vi "create.vi"(9 "Path":string, 10 "Type":enum16{"s3", "gcs"}(ring)) -> (3 "Source":refnum<class "source.lvclass">)   [LabVIEW 2020, in "datasources.lvlib" / "source.lvclass"]
uses:
  source.lvclass
  source.lvclass/source.ctl
  s3/s3.lvclass
  gcs/gcs.lvclass
  C:/code/labview-client/lv_src/Nominal Client/datasources/source/source.lvclass
  C:/code/labview-client/lv_src/Nominal Client/datasources/payload/payload.lvclass
  C:/code/labview-client/lv_src/Nominal Client/datasources/s3/s3.lvclass
  C:/code/labview-client/lv_src/Nominal Client/datasources/gcs/gcs.lvclass
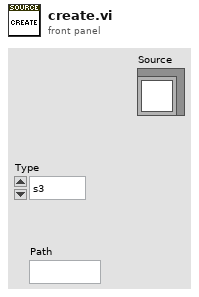
[diagram p1: front panel]
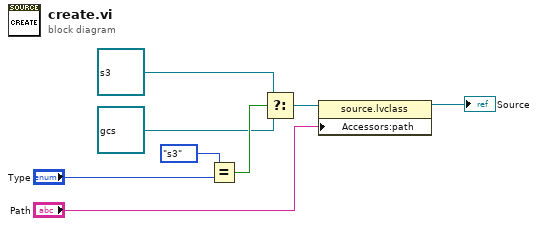
[diagram p0: block diagram]
diagram:
  n1 = Equal?(x=enum16{"s3", "gcs"}."s3", y="Type") -> (x = y?=w7:bool)
  n2 = Select(t=refnum<class "s3.lvclass"> refnum ("datasources.lvlib:s3.lvclass"), s=w7, f=refnum<class "gcs.lvclass"> refnum ("datasources.lvlib:gcs.lvclass")) -> (s? t:f=w4:refnum<class "source.lvclass">)
  n3 = property class="source.lvclass"(reference=w4, "Accessors:path"="Path") -> (reference out=→"Source":refnum<class "source.lvclass">)  [unwired: 1 in, 1 out]
